vi "Read Age Wrapper.vi"(8 "error in (no error)":errorcluster, 11 "myClass in":refnum<class "myClass.lvclass">) -> (0 "error out":errorcluster, 2 "age":dbl, 3 "myClass out":refnum<class "myClass.lvclass">)   [LabVIEW 2013]
uses:
  myClass.lvclass
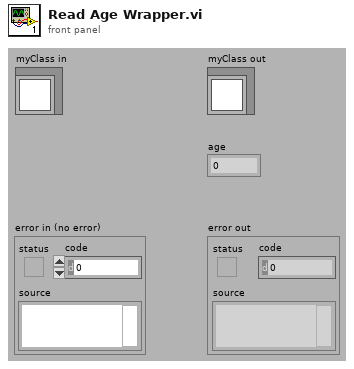
[diagram p1: front panel]
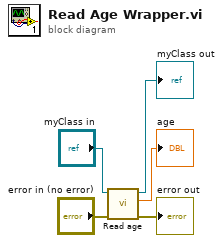
[diagram p0: block diagram]
diagram:
  n1 = call-dynamic "Read age.vi"("error in (no error)"="error in (no error)", "myClass in"="myClass in") -> ("error out"=→"error out":errorcluster, "age"=→"age":dbl, "myClass out"=→"myClass out":refnum<class "myClass.lvclass">)  [unwired: 7 in]
